vi "Test Invalid Write - Bad Flow Name.vi"() -> (2 "Success":bool)   [LabVIEW 2024]
uses:
  Generate Sift Protos/SiftProxy_client/RPC Messages/sift_proxy_v1_ChannelConfig_Flat.ctl
  Generate Sift Protos/SiftProxy_client/RPC Messages/sift_proxy_v1_ChannelDataType.ctl
  Generate Sift Protos/SiftProxy_client/RPC Messages/sift_proxy_v1_ChannelEnumType_Flat.ctl
  Generate Sift Protos/SiftProxy_client/RPC Messages/sift_proxy_v1_ChannelBitFieldElement_Flat.ctl
  Sift API/Sift Client.lvclass
  Generate Sift Protos/SiftProxy_client/SiftProxy_client.lvlib
  Sift Client.lvlib
panel:
  in  "sift_proxy_v1_ChannelConfig_Flat":T1
  out "Error":errorcluster
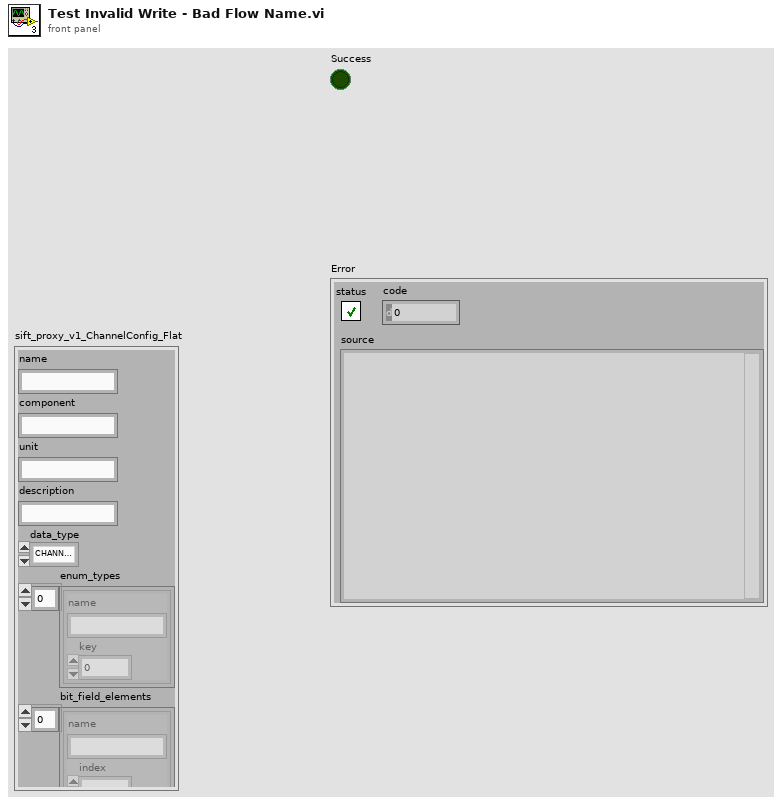
[diagram p1: front panel]
types:
  T1 = typedef "SiftProxy_client.lvlib/sift_proxy_v1_ChannelConfig_Flat.ctl" = cluster{"name":string, "component":string, "unit":string, "description":string, "data_type":T2, "enum_types":T3[], "bit_field_elements":T4[]}
  T2 = typedef "SiftProxy_client.lvlib/sift_proxy_v1_ChannelDataType.ctl" = enum32{"CHANNEL_DATA_TYPE_UNSPECIFIED", "CHANNEL_DATA_TYPE_DOUBLE", "CHANNEL_DATA_TYPE_STRING", "CHANNEL_DATA_TYPE_ENUM", "CHANNEL_DATA_TYPE_BIT_FIELD", "CHANNEL_DATA_TYPE_BOOL", "CHANNEL_DATA_TYPE_FLOAT", "CHANNEL_DATA_TYPE_INT_32", "CHANNEL_DATA_TYPE_UINT_32", "CHANNEL_DATA_TYPE_INT_64", "CHANNEL_DATA_TYPE_UINT_64"}
  T3 = typedef "SiftProxy_client.lvlib/sift_proxy_v1_ChannelEnumType_Flat.ctl" = cluster{"name":string, "key":u32}
  T4 = typedef "SiftProxy_client.lvlib/sift_proxy_v1_ChannelBitFieldElement_Flat.ctl" = cluster{"name":string, "index":i32, "bit_count":u32}
  T5 = typedef "SiftProxy_client.lvlib/google_protobuf_Timestamp.ctl" = cluster{"seconds":i64, "nanos":i32}
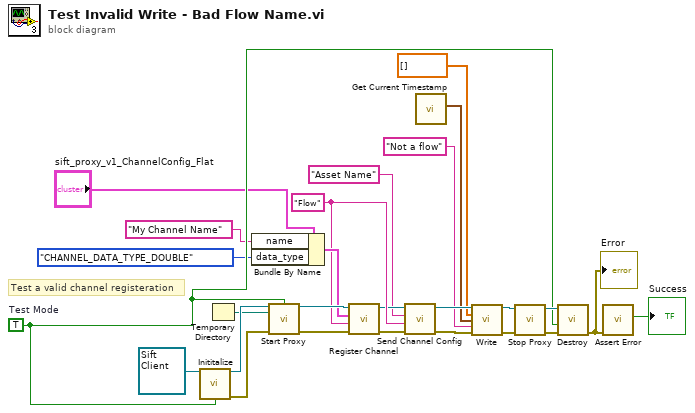
[diagram p0: block diagram]
diagram:
  w13 = "Flow" ("Flow Name")
  w20 = TRUE  # Test Mode
  # "Test a valid channel registeration"
  n1 = call-dynamic "Inititalize.vi"("Sift Client in"=refnum<class "Sift Client.lvclass"> refnum ("Sift Client.lvlib:Sift Client.lvclass"), "Test Mode"=w20) -> ("Sift Client out"=w25:refnum<class "Sift Client.lvclass">, "error out"=w24:errorcluster)  [unwired: 12 in]
  n2 = Temporary Directory() -> (w21:path)
  n3 = Bundle By Name(cluster="sift_proxy_v1_ChannelConfig_Flat", "name"="My Channel Name", "data_type"=sift_proxy_v1_ChannelDataType."CHANNEL_DATA_TYPE_DOUBLE" ("sift_proxy_v1_ChannelDataType")) -> (w15:T1)
  n4 = call-dynamic "Start Proxy.vi"("Sift Client in"=w25, "Test Mode"=w20, "Storage Path"=w21, "error in (no error)"=w24) -> ("Sift Client out"=w19:refnum<class "Sift Client.lvclass">, "error out"=w14:errorcluster)  [unwired: 10 in]
  n5 = call-dynamic "Register Channel.vi"("error in (no error)"=w14, "Flow Name"=w13, "Channel Config"=w15, "Sift Client in"=w19) -> ("error out"=w10:errorcluster, "Sift Client out"=w12:refnum<class "Sift Client.lvclass">)  [unwired: 6 in]
  n6 = call-dynamic "Send Channel Config.vi"("error in (no error)"=w10, "Flow Name"=w13, "Asset Name"="Asset Name", "Sift Client in"=w12) -> ("error out"=w7:errorcluster, "Sift Client out"=w9:refnum<class "Sift Client.lvclass">)  [unwired: 6 in]
  n7 = call "Get Current Timestamp.vi"() -> ("Timestamp"=w5:T5)  [unwired: 11 in]
  n8 = call-dynamic "Write.vi"("Sift Client in"=w9, "Values"=dbl[] [], "Timestamp"=w5, "Flow Name"="Not a flow", "error in (no error)"=w7) -> ("Sift Client out"=w8:refnum<class "Sift Client.lvclass">, "error out"=w6:errorcluster)  [unwired: 9 in]
  n9 = call-dynamic "Stop Proxy.vi"("error in (no error)"=w6, "Sift Client in"=w8) -> ("error out"=w23:errorcluster, "Sift Client out"=w22:refnum<class "Sift Client.lvclass">)  [unwired: 7 in, 1 out]
  n10 = call-dynamic "Destroy.vi"("error in (no error)"=w23, "Test Mode"=w20, "Sift Client in"=w22) -> ("error out"=w2:errorcluster)  [unwired: 7 in, 1 out]
  "Error" <- w2
  n11 = call "Assert Error.vi"("Error"=w2) -> ("Success"=→"Success":bool)  [unwired: 10 in]
